vi "Add Attribute - Timestamp.vi"(6 "UNIX?":bool=TRUE caption="UNIX? (T)", 8 "error in (no error)":errorcluster, 9 "Value":timestamp caption="Value (00:00:00.000 DD/MM/YYYY)", 10 "Attribute":string, 11 "YAML Parser in":refnum<class "YAML Parser.lvclass">) -> (0 "error out":errorcluster, 3 "YAML Parser out":refnum<class "YAML Parser.lvclass">)   [LabVIEW 2015, in "YAML Parser.lvclass"]
uses:
  YAML Parser.lvclass
  YAML Parser.lvclass/YAML Parser.ctl
panel:
  out "replaced":bool
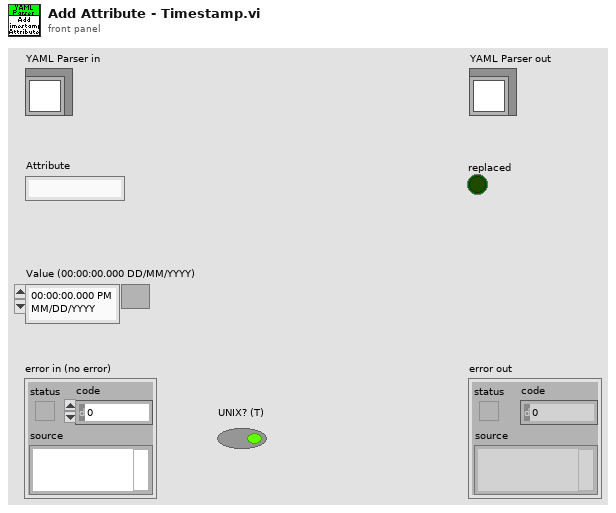
[diagram p1: front panel]
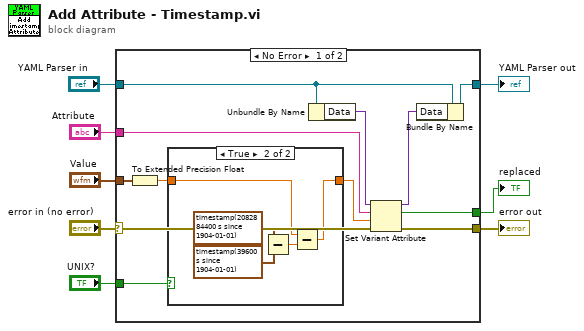
[diagram p0: block diagram]
diagram:
  n1 = case shown="No Error" "error in (no error)" {
    selector: "error in (no error)" -> [w18 w28]
    tunnel: [w17 w28] -> w7
    tunnel: [w20 w27] -> w5
    tunnel: "YAML Parser in" -> [w19 w27]
    tunnel: "Attribute" -> [w14 _]
    tunnel: "Value" -> [w13 _]
    tunnel: [w12 _] -> w2
    tunnel: "UNIX?" -> [w11 _]
    frame No Error {
      n2 = To Extended Precision Float(1:w13) -> (0:w9:ext)
      n3 = case shown="True" w11 {
        tunnel: [w21 w22] -> w10
        tunnel: w9 -> [w21 w23]
        frame False {
        }
        frame True {
          n4 = Subtract(x=timestamp(2082884400 s since 1904-01-01), y=timestamp(39600 s since 1904-01-01)) -> (x-y=w24:dbl)
          n5 = Subtract(x=w23, y=w24) -> (x-y=w22:ext)
        }
      }
      n6 = Unbundle By Name(w19) -> ("Data"=w16:variant)
      n7 = Set Variant Attribute(Variant=w16, name=w14, value=w10, error in=w18) -> (Variant out=w15:variant, replaced=w12:bool, error out=w17:errorcluster)
      n8 = Bundle By Name(cluster=w19, "Data"=w15) -> (w20:refnum<class "YAML Parser.lvclass">)
    }
    frame Error {
    }
  }
  "error out" <- w7
  "YAML Parser out" <- w5
  "replaced" <- w2
